vi "Init.vi"() -> (3 "Nav X Opened?":bool, 4 "Sensors":cluster{T9[], T13[], T14[], T16[]}, 6 "Motors":cluster{T4[]}, 8 "Servos":cluster{T1[]}, 10 "Joysticks":cluster{T18[]}, 14 "NavX":cluster{T20[]} {"?"."navX Common Information"."Update Rate (4Hz-60Hz)" min=4 max=50 step=1; "?"."navX System Information"."Status"."NAVX_OP_STATUS" items=["INITIALIZING", "SELFTEST_IN_PROGRESS", "ERROR", "IMU_AUTOCAL_IN_PROGRESS", "NORMAL"]; "?"."navX System Information"."Status"."NAVX_CAL_STATUS" items=["IMU_CAL_STATE_MASK"=3, "IMU_CAL_INPROGRESS"=0, "IMU_CAL_ACCUMULATE"=1, "IMU_CAL_COMPLETE"=2, "MAG_CAL_COMPLETE"=4, "BARO_CAL_COMPLETE"=8]; "?"."navX Interface Protocol TypeDefs"."I2CDevRef"."Device Address" format="%.0x"}, 15 "Nav X Error":errorcluster)   [LabVIEW 2015]
uses:
  Peripherals/Buzz XXI Peripherals/Nav X Library/navX-MXP Library/COMMON/TypeDefs/navX Device TypeDef.ctl
  Peripherals/Buzz XXI Peripherals/Nav X Library/navX-MXP Library/COMMON/TypeDefs/Value TypeDefs/navX Interface Protocol.ctl
  <vilib>/Rock Robotics/WPI/SPI/WPI_SPIDevRef.ctl
  <vilib>/Rock Robotics/SystemInterfaces/spilib/spi_bus.ctl
  <vilib>/Rock Robotics/WPI/I2C/WPI_I2CDevRef.ctl
  <vilib>/Rock Robotics/SystemInterfaces/i2clib/i2c_bus.ctl
  Peripherals/Buzz XXI Peripherals/Nav X Library/navX-MXP Library/COMMON/TypeDefs/Data TypeDefs/navX Board Information.ctl
  Peripherals/Buzz XXI Peripherals/Nav X Library/navX-MXP Library/COMMON/TypeDefs/Data TypeDefs/navX Status Data.ctl
  Peripherals/Buzz XXI Peripherals/Nav X Library/navX-MXP Library/COMMON/TypeDefs/Value TypeDefs/navX NAVX_OP_STATUS.ctl
  Peripherals/Buzz XXI Peripherals/Nav X Library/navX-MXP Library/COMMON/TypeDefs/Value TypeDefs/navX NAVX_CAL_STATUS.ctl
  Peripherals/Buzz XXI Peripherals/Nav X Library/navX-MXP Library/COMMON/TypeDefs/Value TypeDefs/navX NAVX_SENSOR_STATUS.ctl
  Peripherals/Buzz XXI Peripherals/Nav X Library/navX-MXP Library/COMMON/TypeDefs/Data TypeDefs/navX Offsets Data.ctl
  Peripherals/Buzz XXI Peripherals/Nav X Library/navX-MXP Library/COMMON/TypeDefs/Value TypeDefs/navX Update Rate.ctl
  <vilib>/Rock Robotics/WPI/Joystick/WPI_JoystickDevRef.ctl
  <vilib>/Rock Robotics/WPI/Joystick/WPI_JoystickDeviceEnum.ctl
  <vilib>/Rock Robotics/WPI/Encoder/WPI_EncoderDevRef.ctl
  <vilib>/Rock Robotics/SystemInterfaces/Encoder/FPGA_EncoderIdx.ctl
  <vilib>/Rock Robotics/SystemInterfaces/Counter/FPGA_CounterCtrSystemIndex.ctl
  <vilib>/Rock Robotics/WPI/Encoder/WPI_EncoderType.ctl
  <vilib>/Rock Robotics/WPI/Counter/WPI_CounterDevRef.ctl
  <vilib>/Rock Robotics/WPI/Switch/WPI_SwitchDevRef.ctl
  <vilib>/Rock Robotics/SystemInterfaces/DIO/FPGA_DIOChannel.ctl
  <vilib>/Rock Robotics/WPI/Potentiometer/WPI_PotentiometerDevRef.ctl
  <vilib>/Rock Robotics/SystemInterfaces/AI/FPGA_AIChannel.ctl
  <vilib>/Rock Robotics/WPI/MotorControl/WPI_MotorControlDeviceRef.ctl
  <vilib>/Rock Robotics/WPI/MotorControl/WPI_MotorControlType.ctl
  <vilib>/Rock Robotics/SystemInterfaces/DIO/FPGA_DIOPWMChannel.ctl
  <vilib>/Rock Robotics/WPI/PWM/WPI_PWMDeadband.ctl
  <vilib>/Rock Robotics/WPI/CAN/Jaguar/SubVIs/WPI_CANJaguar_ControlMode.ctl
  <vilib>/Rock Robotics/WPI/CAN/TalonSRX/WPI_CANTalonSRX_APIControlMode.ctl
  <vilib>/Rock Robotics/WPI/PWM/Servo/WPI_ServoDeviceRef.ctl
  <vilib>/Rock Robotics/WPI/MotorControl/WPI_MotorControlOpenCANTalonSRX.vi
  <vilib>/Rock Robotics/WPI/Counter/WPI_CounterDigitalInputToDigitalSource.vi
  <vilib>/Rock Robotics/WPI/Counter/WPI_CounterOpen UpDown Mode.vi
  <vilib>/Rock Robotics/WPI/Switch/WPI_SwitchOpenLimit.vi
  Peripherals/Buzz XXI Peripherals/Nav X Library/navX-MXP Library/navX-MXP IMU.lvlib
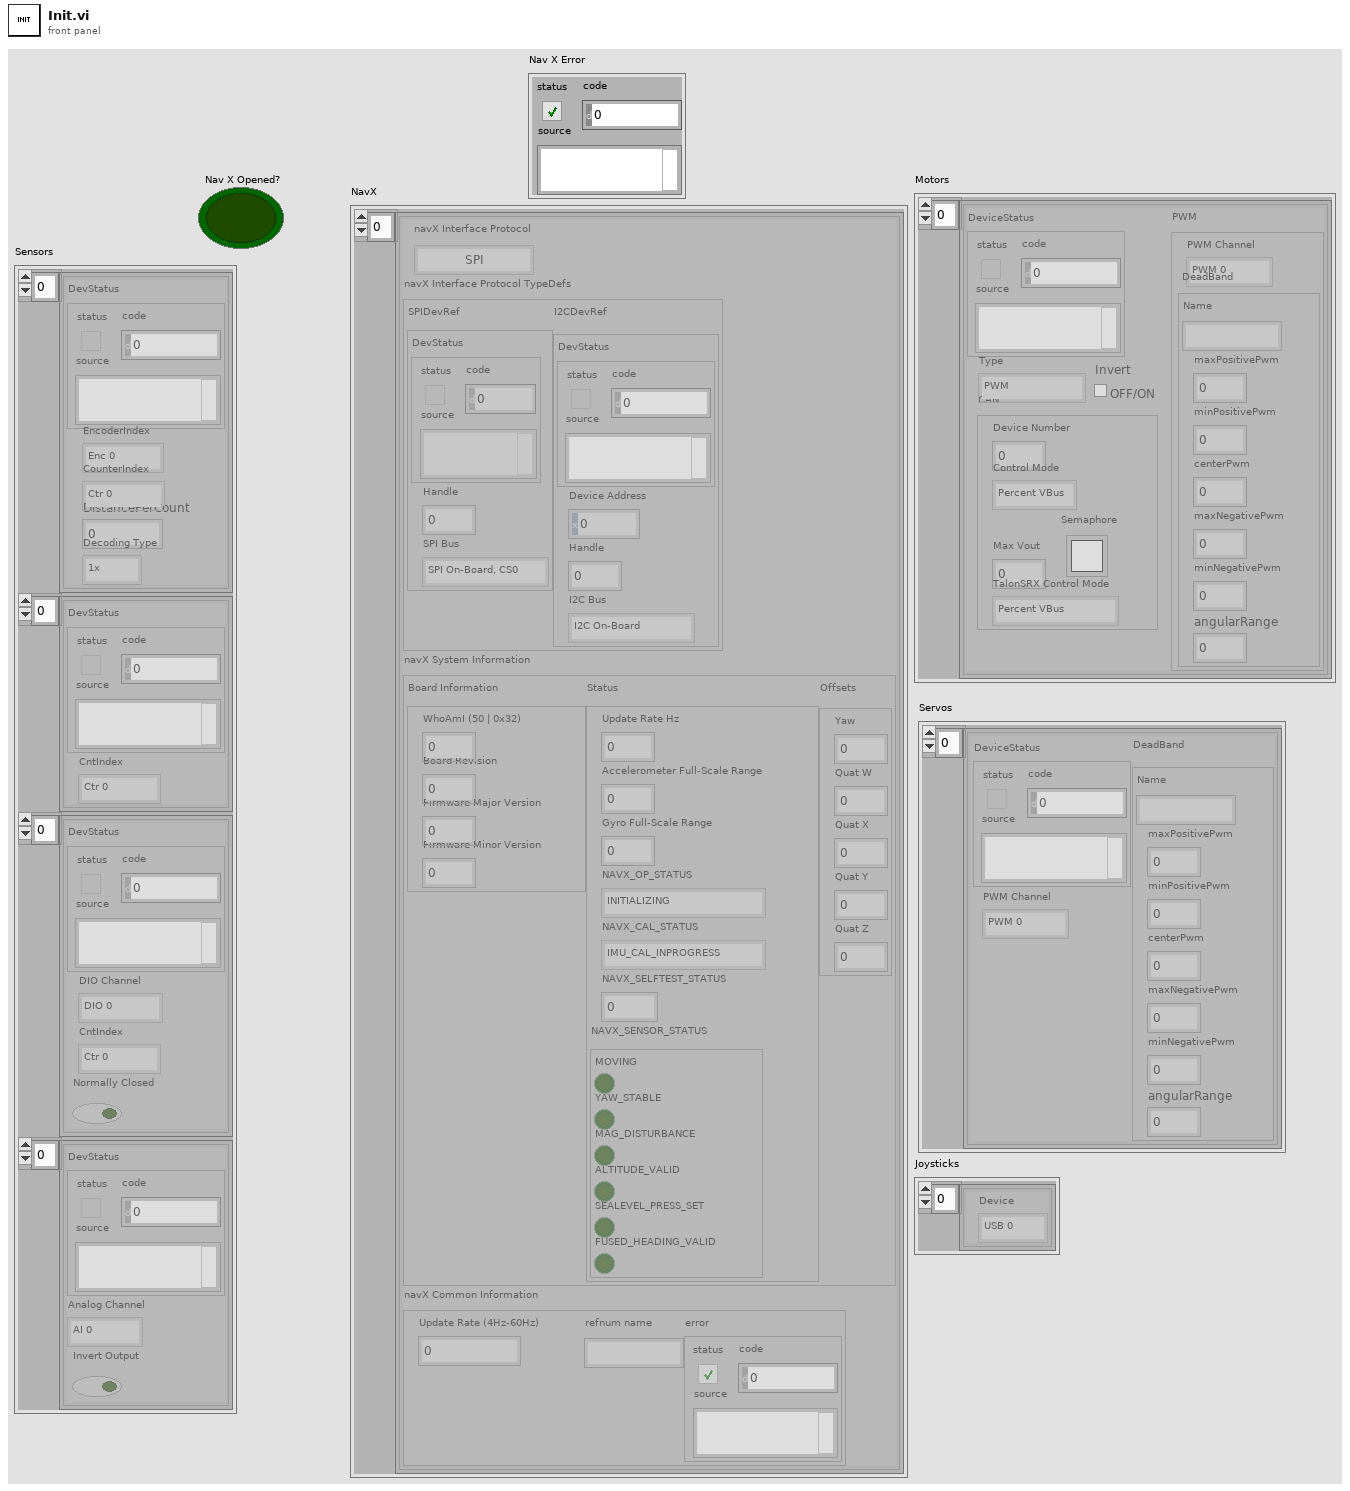
[diagram p1: front panel]
types:
  T1 = typedef "WPI_ServoDeviceRef.ctl" = cluster{"DeviceStatus":errorcluster, "PWM Channel":T2, "DeadBand":T3}
  T2 = typedef "FPGA_DIOPWMChannel.ctl" = enum8{"PWM 0", "PWM 1", "PWM 2", "PWM 3", "PWM 4", "PWM 5", "PWM 6", "PWM 7", "PWM 8", "PWM 9", "PWM MXP 0", "PWM MXP 1", "PWM MXP 2", "PWM MXP 3", "PWM MXP 4", "PWM MXP 5", "PWM MXP 6", "PWM MXP 7", "PWM MXP 8", "PWM MXP 9", "Invalid"}
  T3 = typedef "WPI_PWMDeadband.ctl" = cluster{"Name":string, "maxPositivePwm":i32, "minPositivePwm":i32, "centerPwm":i32, "maxNegativePwm":i32, "minNegativePwm":i32, "angularRange":u16}
  T4 = typedef "WPI_MotorControlDeviceRef.ctl" = cluster{"DeviceStatus":errorcluster, "Type":T5, "PWM":cluster{"PWM Channel":T2, "DeadBand":T3}, "CAN":cluster{"Device Number":u8, "Control Mode":T6, "Semaphore":T7, "Max Vout":dbl, "TalonSRX Control Mode":T8}, "Invert":bool}
  T5 = typedef "WPI_MotorControlType.ctl" = enum16{"PWM", "CAN", "CANTalonSRX"}
  T6 = typedef "WPI_CANJaguar_ControlMode.ctl" = enum8{"Percent VBus", "Current", "Speed", "Position", "Voltage"}
  T7 = typedef "Semaphore RefNum" = refnum<k1>
  T8 = typedef "WPI_CANTalonSRX_APIControlMode.ctl" = enum8{"Percent VBus", "Speed", "Position", "Slave", "Unchanged / Invalid", "Voltage Compensation", "Current", "Motion Profile"}
  T9 = typedef "WPI_EncoderDevRef.ctl" = cluster{"DevStatus":errorcluster, "EncoderIndex":T10, "CounterIndex":T11, "DistancePerCount":dbl, "Decoding Type":T12}
  T10 = typedef "FPGA_EncoderIdx.ctl" = enum8{"Enc 0", "Enc 1", "Enc 2", "Enc 3", "Enc 4", "Enc 5", "Enc 6", "Enc 7", "Invalid"}
  T11 = typedef "FPGA_CounterCtrSystemIndex.ctl" = enum8{"Ctr 0", "Ctr 1", "Ctr 2", "Ctr 3", "Ctr 4", "Ctr 5", "Ctr 6", "Ctr 7", "Invalid"}
  T12 = typedef "WPI_EncoderType.ctl" = enum16{"1x", "2x", "4x"}
  T13 = typedef "WPI_CounterDevRef.ctl" = cluster{"DevStatus":errorcluster, "CntIndex":T11}
  T14 = typedef "WPI_SwitchDevRef.ctl" = cluster{"DevStatus":errorcluster, "DIO Channel":T15, "CntIndex":T11, "Normally Closed":bool}
  T15 = typedef "FPGA_DIOChannel.ctl" = enum8{"DIO 0", "DIO 1", "DIO 2", "DIO 3", "DIO 4", "DIO 5", "DIO 6", "DIO 7", "DIO 8", "DIO 9", "DIO MXP 0", "DIO MXP 1", "DIO MXP 2", "DIO MXP 3", "DIO MXP 4", "DIO MXP 5", "DIO MXP 6", "DIO MXP 7", "DIO MXP 8", "DIO MXP 9", "DIO MXP 10", "DIO MXP 11", "DIO MXP 12", "DIO MXP 13", "DIO MXP 14", "DIO MXP 15", "Invalid"}
  T16 = typedef "WPI_PotentiometerDevRef.ctl" = cluster{"DevStatus":errorcluster, "Analog Channel":T17, "Invert Output":bool}
  T17 = typedef "FPGA_AIChannel.ctl" = enum8{"AI 0", "AI 1", "AI 2", "AI 3", "AI MXP 0", "AI MXP 1", "AI MXP 2", "AI MXP 3", "Invalid"}
  T18 = typedef "WPI_JoystickDevRef.ctl" = cluster{"Device":T19}
  T19 = typedef "WPI_JoystickDeviceEnum.ctl" = enum16{"USB 0", "USB 1", "USB 2", "USB 3", "USB 4", "USB 5"}
  T20 = typedef "navX-MXP IMU.lvlib/navX Device TypeDef.ctl" = cluster{"navX Interface Protocol":T21, "navX Interface Protocol TypeDefs":cluster{"SPIDevRef":T22, "I2CDevRef":T24}, "navX System Information":cluster{"Board Information":T26, "Status":T27, "Offsets":T31}, "navX Common Information":cluster{"Update Rate (4Hz-60Hz)":T32, "refnum name":string, "error":errorcluster}}
  T21 = typedef "navX-MXP IMU.lvlib/navX Interface Protocol.ctl" = enum16{"SPI", "I2C"}
  T22 = typedef "WPI_SPIDevRef.ctl" = cluster{"DevStatus":errorcluster, "Handle":i32, "SPI Bus":T23}
  T23 = typedef "spi_bus.ctl" = enum16{"SPI On-Board, CS0", "SPI On-Board, CS1", "SPI On-Board, CS2", "SPI On-Board, CS3", "SPI MXP", "Invalid"}
  T24 = typedef "WPI_I2CDevRef.ctl" = cluster{"DevStatus":errorcluster, "Device Address":u8, "Handle":i32, "I2C Bus":T25}
  T25 = typedef "i2c_bus.ctl" = enum16{"I2C On-Board", "I2C MXP", "Invalid"}
  T26 = typedef "navX-MXP IMU.lvlib/navX Board Information.ctl" = cluster{"WhoAmI (50 | 0x32)":u8, "Board Revision":u8, "Firmware Major Version":u8, "Firmware Minor Version":u8}
  T27 = typedef "navX-MXP IMU.lvlib/navX Status Data.ctl" = cluster{"Update Rate Hz":u8, "Accelerometer Full-Scale Range":u8, "Gyro Full-Scale Range":u16, "NAVX_OP_STATUS":T28, "NAVX_CAL_STATUS":T29, "NAVX_SELFTEST_STATUS":u8, "NAVX_SENSOR_STATUS":T30}
  T28 = typedef "navX-MXP IMU.lvlib/navX NAVX_OP_STATUS.ctl" = u8
  T29 = typedef "navX-MXP IMU.lvlib/navX NAVX_CAL_STATUS.ctl" = u8
  T30 = typedef "navX-MXP IMU.lvlib/navX NAVX_SENSOR_STATUS.ctl" = cluster{"MOVING":bool, "YAW_STABLE":bool, "MAG_DISTURBANCE":bool, "ALTITUDE_VALID":bool, "SEALEVEL_PRESS_SET":bool, "FUSED_HEADING_VALID":bool}
  T31 = typedef "navX-MXP IMU.lvlib/navX Offsets Data.ctl" = cluster{"Yaw":dbl, "Quat W":dbl, "Quat X":dbl, "Quat Y":dbl, "Quat Z":dbl}
  T32 = typedef "navX-MXP IMU.lvlib/navX Update Rate.ctl" = u8
  T33 = typedef "WPI_DigitalInputDevRef.ctl" = cluster{"DevStatus":errorcluster, "DIO Channel":T15}
  T34 = typedef "FPGA_CounterEncoderSourceConvertionLVSourceType.ctl" = cluster{"DevStatus":errorcluster, "AnalogTriggerMode?":bool, "DigitalMode":cluster{"DIO Channel":T35}, "AnalogTriggerMode":cluster{"AnalogTriggerIndex":T36, "OutputType":T37}}
  T35 = typedef "FPGA_DIODigitalSourceChannel.ctl" = enum8{"DIO 0", "DIO 1", "DIO 2", "DIO 3", "DIO 4", "DIO 5", "DIO 6", "DIO 7", "DIO 8", "DIO 9", "DIO MXP 0", "DIO MXP 1", "DIO MXP 2", "DIO MXP 3", "DIO MXP 4", "DIO MXP 5", "DIO MXP 6", "DIO MXP 7", "DIO MXP 8", "DIO MXP 9", "DIO MXP 10", "DIO MXP 11", "DIO MXP 12", "DIO MXP 13", "DIO MXP 14", "DIO MXP 15", "Disabled"}
  T36 = typedef "FPGA_AnalogTriggerIndex.ctl" = enum8{"Trig 0", "Trig 1", "Trig 2", "Trig 3", "Trig 4", "Trig 5", "Trig 6", "Trig 7", "Invalid"}
  T37 = typedef "FPGA_AnalogTriggerOutType.ctl" = enum16{"InWindow", "TriggerState", "Rising", "Falling"}
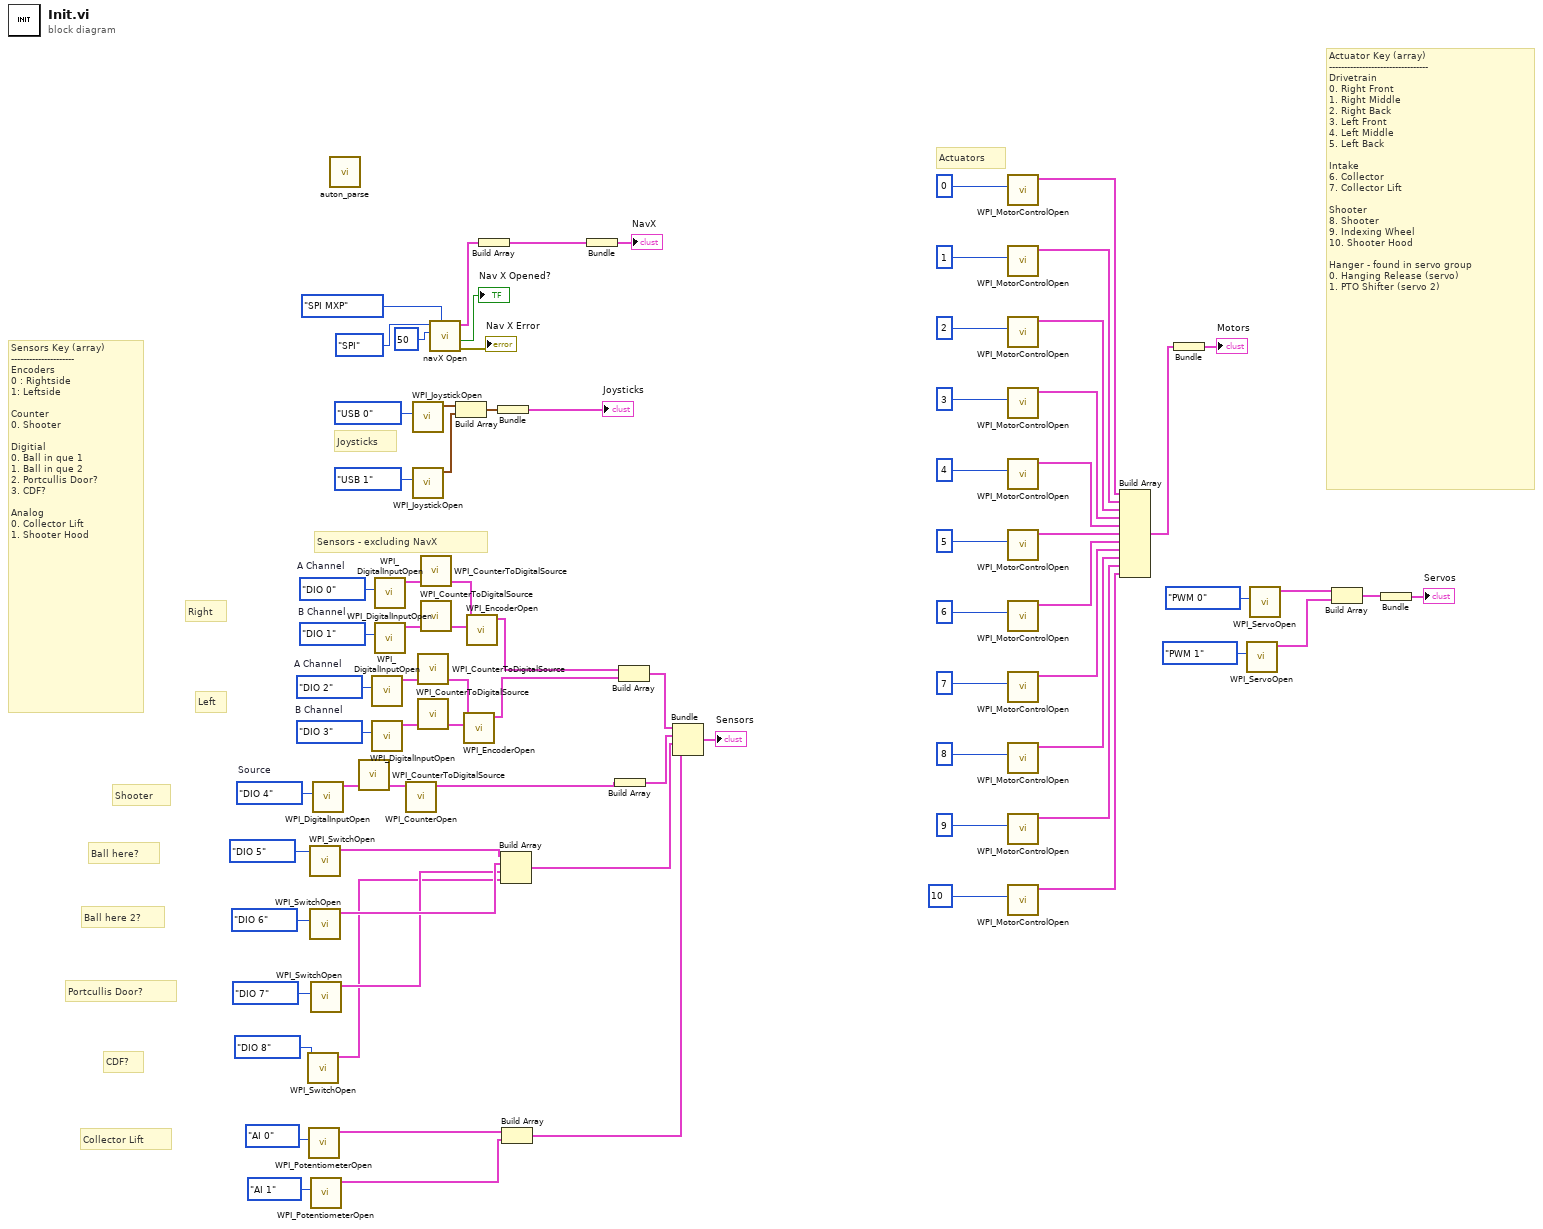
[diagram p0: block diagram]
diagram:
  w14 = FPGA_DIOChannel."DIO 4"  # Source
  w21 = FPGA_DIOChannel."DIO 3"  # B Channel
  w20 = FPGA_DIOChannel."DIO 2"  # A Channel
  w27 = FPGA_DIOChannel."DIO 1"  # B Channel
  w26 = FPGA_DIOChannel."DIO 0"  # A Channel
  # "Sensors - excluding NavX"
  # "Actuators"
  # "CDF?"
  # "Portcullis Door?"
  # "Ball here 2?"
  # "Collector Lift"
  # "Ball here?"
  # "Shooter"
  # "Left"
  # "Right"
  # "Sensors Key (array)\n---------------------\nEncoders\n0 : Rightside\n1: Leftside\n\nCounter\n0. Shooter\n\nDigitial\n0. Ball in que 1\n1. Ball in que 2\n2. Portcullis Door?\n3. CDF?\n\nAnalog\n0. Collector Lift\n1. Shooter Hood"
  # "Actuator Key (array)\n--------------------------------- \nDrivetrain\n0. Right Front\n1. Right Middle\n2. Right Back\n3. Left Front\n4. Left Middle\n5. Left Back\n\nIntake\n6. Collector\n7. Collector Lift\n\nShooter\n8. Shooter\n9. Indexing Wheel\n10. Shooter Hood\n\nHanger - found in servo group\n0. Hanging Release (servo)\n1. PTO Shifter (servo 2)"
  # "Joysticks"
  n1 = call-poly <vilib>:"WPI_SwitchOpen.vi"("DIO Channel"=FPGA_DIOChannel."DIO 8") -> ("SwitchDevRef"=w3:T14)  [unwired: 9 in, 1 out]
  n2 = call <vilib>:"WPI_PotentiometerOpen.vi"("Analog Channel"=FPGA_AIChannel."AI 0") -> ("PotDevRef"=w11:T16)  [unwired: 9 in, 1 out]
  n3 = call-poly <vilib>:"WPI_SwitchOpen.vi"("DIO Channel"=FPGA_DIOChannel."DIO 5") -> ("SwitchDevRef"=w9:T14)  [unwired: 9 in, 1 out]
  n4 = call-poly <vilib>:"WPI_SwitchOpen.vi"("DIO Channel"=FPGA_DIOChannel."DIO 6") -> ("SwitchDevRef"=w5:T14)  [unwired: 9 in, 1 out]
  n5 = call-poly <vilib>:"WPI_SwitchOpen.vi"("DIO Channel"=FPGA_DIOChannel."DIO 7") -> ("SwitchDevRef"=w4:T14)  [unwired: 9 in, 1 out]
  n6 = call <vilib>:"WPI_PotentiometerOpen.vi"("Analog Channel"=FPGA_AIChannel."AI 1") -> ("PotDevRef"=w1:T16)  [unwired: 9 in, 1 out]
  n7 = call <vilib>:"WPI_DigitalInputOpen.vi"("DIO Channel"=w14) -> ("DigitalInputDevRef"=w13:T33)  [unwired: 1 in, 9 out]
  n8 = call "auton_parse.vi"() -> ()  [unwired: 1 in]
  n9 = call-poly <vilib>:"WPI_CounterToDigitalSource.vi"("DigitalInputDevRef"=w13) -> ("Digital Source"=w15:T34)  [unwired: 6 out]
  n10 = call <vilib>:"WPI_DigitalInputOpen.vi"("DIO Channel"=w20) -> ("DigitalInputDevRef"=w17:T33)  [unwired: 1 in, 9 out]
  n11 = call <vilib>:"WPI_DigitalInputOpen.vi"("DIO Channel"=w21) -> ("DigitalInputDevRef"=w18:T33)  [unwired: 1 in, 9 out]
  n12 = call <vilib>:"WPI_DigitalInputOpen.vi"("DIO Channel"=w26) -> ("DigitalInputDevRef"=w23:T33)  [unwired: 1 in, 9 out]
  n13 = call <vilib>:"WPI_DigitalInputOpen.vi"("DIO Channel"=w27) -> ("DigitalInputDevRef"=w24:T33)  [unwired: 1 in, 9 out]
  n14 = call-poly <vilib>:"WPI_CounterOpen.vi"("Up Source"=w15) -> ("CounterDevRef"=w68:T13)  [unwired: 6 in, 4 out]
  n15 = call <vilib>:"WPI_JoystickOpen.vi"("JoystickDevice"=WPI_JoystickDeviceEnum."USB 0") -> ("JoystickDevRef"=w75:T18)  [unwired: 10 in]
  n16 = call <vilib>:"WPI_JoystickOpen.vi"("JoystickDevice"=WPI_JoystickDeviceEnum."USB 1") -> ("JoystickDevRef"=w74:T18)  [unwired: 10 in]
  n17 = call-poly <vilib>:"WPI_CounterToDigitalSource.vi"("DigitalInputDevRef"=w17) -> ("Digital Source"=w16:T34)  [unwired: 6 out]
  n18 = call-poly <vilib>:"WPI_CounterToDigitalSource.vi"("DigitalInputDevRef"=w18) -> ("Digital Source"=w19:T34)  [unwired: 6 out]
  n19 = call-poly <vilib>:"WPI_CounterToDigitalSource.vi"("DigitalInputDevRef"=w23) -> ("Digital Source"=w22:T34)  [unwired: 6 out]
  n20 = call-poly <vilib>:"WPI_CounterToDigitalSource.vi"("DigitalInputDevRef"=w24) -> ("Digital Source"=w25:T34)  [unwired: 6 out]
  n21 = call "navX Open.vi"("SPI Bus"=spi_bus."SPI MXP", "Update Rate (4Hz-60Hz)"=T32 50, "navX Interface Protocol"=navX_Interface_Protocol."SPI") -> ("error out"=→"Nav X Error":errorcluster, "Opened?"=→"Nav X Opened?":bool, "navX Device TypeDef"=w55:T20)  [unwired: 6 in]
  n22 = Build Array(w75, w74) -> (w73:T18[])
  n23 = call <vilib>:"WPI_EncoderOpen.vi"("BSource"=w19, "ASource"=w16) -> ("EncoderDevRef"=w69:T9)  [unwired: 6 in, 3 out]
  n24 = call <vilib>:"WPI_EncoderOpen.vi"("BSource"=w25, "ASource"=w22) -> ("EncoderDevRef"=w70:T9)  [unwired: 6 in, 3 out]
  n25 = Build Array(w55) -> (w79:T20[])
  n26 = Bundle(w73) -> (→"Joysticks":cluster{T18[]})  [unwired: 1 in]
  n27 = Build Array(w9, w5, w4, w3) -> (w65:T14[])
  n28 = Build Array(w11, w1) -> (w64:T16[])
  n29 = Bundle(w79) -> (→"NavX":cluster{T20[]})  [unwired: 1 in]
  n30 = Build Array(w68) -> (w67:T13[])
  n31 = Build Array(w70, w69) -> (w66:T9[])
  n32 = Bundle(w66, w67, w65, w64) -> (→"Sensors":cluster{T9[], T13[], T14[], T16[]})  [unwired: 1 in]
  n33 = call-poly <vilib>:"WPI_MotorControlOpen.vi"("Device Number"=u8 0) -> ("MotorControlDeviceRef"=w47:T4)  [unwired: 9 in, 1 out]
  n34 = call-poly <vilib>:"WPI_MotorControlOpen.vi"("Device Number"=u8 1) -> ("MotorControlDeviceRef"=w46:T4)  [unwired: 9 in, 1 out]
  n35 = call-poly <vilib>:"WPI_MotorControlOpen.vi"("Device Number"=u8 2) -> ("MotorControlDeviceRef"=w45:T4)  [unwired: 9 in, 1 out]
  n36 = call-poly <vilib>:"WPI_MotorControlOpen.vi"("Device Number"=u8 3) -> ("MotorControlDeviceRef"=w44:T4)  [unwired: 9 in, 1 out]
  n37 = call-poly <vilib>:"WPI_MotorControlOpen.vi"("Device Number"=u8 4) -> ("MotorControlDeviceRef"=w43:T4)  [unwired: 9 in, 1 out]
  n38 = call-poly <vilib>:"WPI_MotorControlOpen.vi"("Device Number"=5) -> ("MotorControlDeviceRef"=w42:T4)  [unwired: 9 in, 1 out]
  n39 = call-poly <vilib>:"WPI_MotorControlOpen.vi"("Device Number"=u8 6) -> ("MotorControlDeviceRef"=w37:T4)  [unwired: 9 in, 1 out]
  n40 = call-poly <vilib>:"WPI_MotorControlOpen.vi"("Device Number"=u8 7) -> ("MotorControlDeviceRef"=w36:T4)  [unwired: 9 in, 1 out]
  n41 = call-poly <vilib>:"WPI_MotorControlOpen.vi"("Device Number"=u8 8) -> ("MotorControlDeviceRef"=w35:T4)  [unwired: 9 in, 1 out]
  n42 = call-poly <vilib>:"WPI_MotorControlOpen.vi"("Device Number"=u8 9) -> ("MotorControlDeviceRef"=w34:T4)  [unwired: 9 in, 1 out]
  n43 = call-poly <vilib>:"WPI_MotorControlOpen.vi"("Device Number"=10) -> ("MotorControlDeviceRef"=w32:T4)  [unwired: 9 in, 1 out]
  n44 = Build Array(w47, w46, w45, w44, w43, w42, w37, w36, w35, w34, w32) -> (w71:T4[])
  n45 = Bundle(w71) -> (→"Motors":cluster{T4[]})  [unwired: 1 in]
  n46 = call <vilib>:"WPI_ServoOpen.vi"("PWM Channel"=FPGA_DIOPWMChannel."PWM 1") -> ("ServoDeviceRef"=w28:T1)  [unwired: 9 in, 1 out]
  n47 = call <vilib>:"WPI_ServoOpen.vi"("PWM Channel"=FPGA_DIOPWMChannel."PWM 0") -> ("ServoDeviceRef"=w29:T1)  [unwired: 9 in, 1 out]
  n48 = Build Array(w29, w28) -> (w62:T1[])
  n49 = Bundle(w62) -> (→"Servos":cluster{T1[]})  [unwired: 1 in]
